vi "Create.vi"(9 "Queue Actor":refnum<class "Queue Actor.lvclass">, 10 "Alias":string, 11 "jettl Queue Actor in":refnum<class "jettl Queue Actor.lvclass">) -> (3 "jettl Queue Actor out":refnum<class "jettl Queue Actor.lvclass">)   [LabVIEW 2021, in "jettl Queue Actor.lvlib" / "jettl Queue Actor.lvclass"]
uses:
  jettl Queue Actor.lvclass
  Actor/Msg/Msg.lvclass
  Actor/Queue Actor/Queue Actor.lvclass
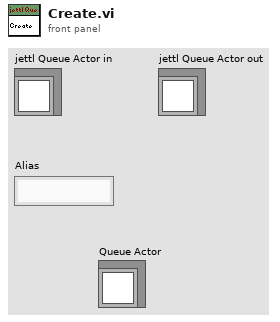
[diagram p1: front panel]
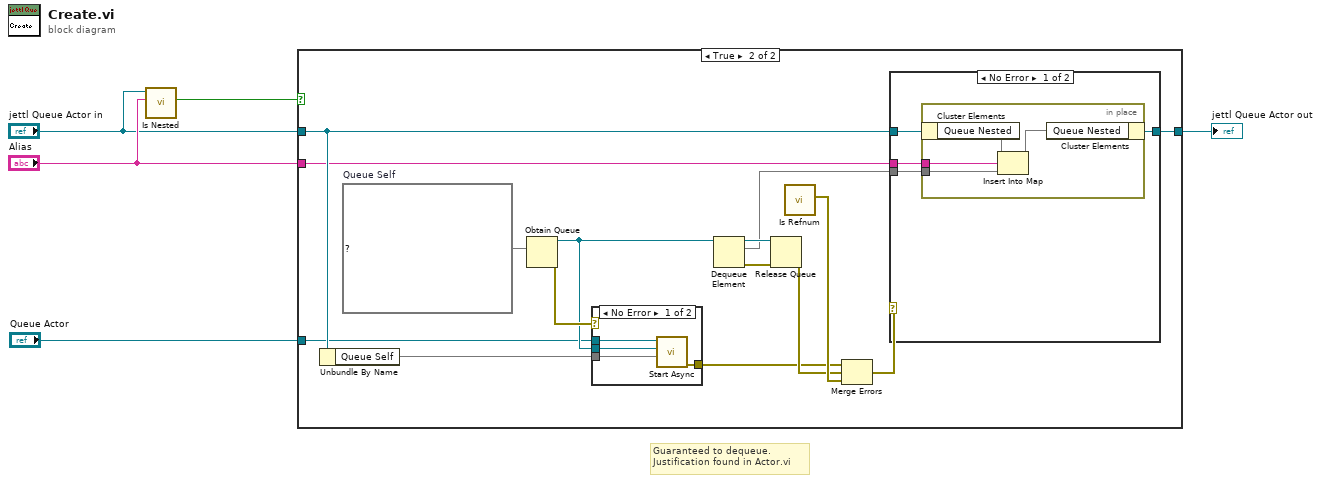
[diagram p0: block diagram]
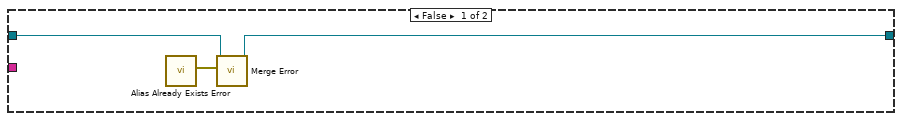
[diagram p2: hidden frame]
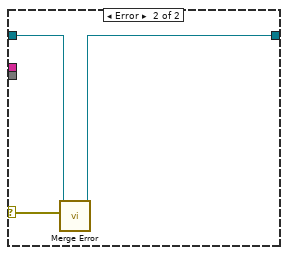
[diagram p4: hidden frame]
diagram:
  # "Guaranteed to dequeue. Justification found in Actor.vi"
  n1 = call-dynamic "Is Nested.vi"("Alias"="Alias", "jettl Queue Actor in"="jettl Queue Actor in") -> ("Nested?"=w3:bool)  [unwired: 9 in]
  n2 = case shown="True" w3 {
    tunnel: "Queue Actor" -> [_ w9]
    tunnel: "jettl Queue Actor in" -> [w8 w18]
    tunnel: "Alias" -> [_ w17]
    tunnel: [w7 w16] -> w4
    frame False {
      n3 = call "Alias Already Exists Error.vi"() -> ("Error"=w6:errorcluster)  [unwired: 11 in]
      n4 = call-dynamic "Merge Error.vi"("Error"=w6, "jettl Queue Actor in"=w8) -> ("jettl Queue Actor out"=w7:refnum<class "jettl Queue Actor.lvclass">)  [unwired: 9 in]
    }
    frame True {
      w11 = map{string, refnum<data-value>} {}  # Queue Self
      n5 = Unbundle By Name(w18) -> ("Queue Self"=w19:map{string, refnum<data-value>})
      n6 = Obtain Queue(element data type=w11) -> (queue out=w10:refnum<queue>, error out=w23:errorcluster)  [unwired: 4 in, 1 out]
      n7 = case shown="No Error" w23 {
        selector: w23 -> [_ w28]
        tunnel: [w26 w28] -> w12
        tunnel: w9 -> [w27 _]
        tunnel: w19 -> [w24 _]
        tunnel: w10 -> [w25 _]
        frame No Error {
          n8 = call "Start Async.vi"("Queue Caller"=w24, "Queue of Queue Self"=w25, "Queue Actor"=w27) -> ("error out"=w26:errorcluster)  [unwired: 8 in]
        }
        frame Error {
        }
      }
      n9 = Dequeue Element(queue=w10) -> (queue out=w21:refnum<queue>, element=w15:map{string, refnum<data-value>}, error out=w22:errorcluster)  [unwired: 2 in, 1 out]
      n10 = Release Queue(queue=w21, error in (no error)=w22) -> (error out=w13:errorcluster)  [unwired: 1 in, 2 out]
      n11 = call "Is Refnum.vi"() -> ("Error"=w14:errorcluster)  [unwired: 11 in]
      n12 = Merge Errors(w12, w13, w14) -> (w20:errorcluster)
      n13 = case shown="No Error" w20 {
        selector: w20 -> [_ w37]
        tunnel: w18 -> [w32 w39]
        tunnel: [w31 w38] -> w16
        tunnel: w15 -> [w30 _]
        tunnel: w17 -> [w29 _]
        frame No Error {
          n14 = in-place {
            in-place-border: w30 -> [w34]
            in-place-border: w29 -> [w33]
            n15 = in-place-cluster #1(w32) -> ("Queue Nested"=w36:map{string, refnum<data-value>})
            n16 = Insert Into Map(map in=w36, key=w33, value=w34) -> (map out=w35:map{string, refnum<data-value>})  [unwired: 2 out]
            n17 = in-place-cluster #1("Queue Nested"=w35) -> (w31:refnum<class "jettl Queue Actor.lvclass">)
          }
        }
        frame Error {
          n18 = call-dynamic "Merge Error.vi"("Error"=w37, "jettl Queue Actor in"=w39) -> ("jettl Queue Actor out"=w38:refnum<class "jettl Queue Actor.lvclass">)  [unwired: 9 in]
        }
      }
    }
  }
  "jettl Queue Actor out" <- w4
